vi "LVObject to JSON - Non Serializable Class - Returns Empty String.vi"() -> ()   [LabVIEW 2017, in "JSON Serializable Serializer Tests.lvlib"]
uses:
  JSON Serializable Serializer Tests.lvlib
  JSON Serializable Serializer/JSON Serializable Serializer.lvclass
  <vilib>/addons/_JKI Toolkits/Caraya/classes/Assert/Assert Equal Value_Variant.vi
  <vilib>/addons/_JKI Toolkits/Caraya/classes/Test/Test.lvclass
  <vilib>/addons/_JKI Toolkits/Caraya/classes/Assert/Assert.lvclass
panel:
  out "error out":errorcluster
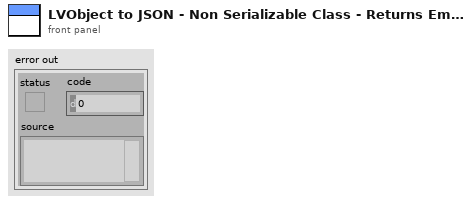
[diagram p1: front panel]
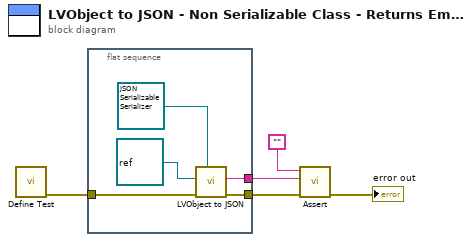
[diagram p0: block diagram]
diagram:
  n1 = call <vilib>:"Define Test.vi"() -> ("error out"=w3:errorcluster)  [unwired: 11 in]
  n2 = flat-sequence {
    tunnel: [w6] -> w5
    tunnel: [w7] -> w4
    tunnel: w3 -> [w8]
    frame #0 {
      n3 = call-dynamic "LVObject to JSON.vi"("JSON Serializer in"=refnum<class "JSON Serializable Serializer.lvclass"> refnum ("JSON Serializer.lvclass"), "error in (no error)"=w8, "Object"=refnum<class> refnum ("Type")) -> ("error out"=w7:errorcluster, "<JSON>Object"=w6:string)  [unwired: 7 in]
    }
  }
  n4 = call-poly <vilib>:"Assert.vi"("error in (no error)"=w4, "Y"=w5, "X"="") -> ("error out"=→"error out":errorcluster)  [unwired: 8 in]
